vi "Fetch Measurement (Adjacent Channel Power Ratio).vi"(0 "VISA resource name":refnum<visa-resource-name>, 11 "error in (no error)":errorcluster) -> (3 "Main Channel Power(dBm)":dbl, 4 "VISA resource name out":refnum<visa-resource-name>, 6 "Low Adjacent Channel Power(dBm)":dbl[](array[numeric]), 8 "Upper Adjacent Channel Power Ratio(dB)":dbl[](array[numeric]), 10 "Low Adjacent Channel Power Ratio(dB)":dbl[](array[numeric]), 14 "Upper Adjacent Channel Power(dBm)":dbl[](array[numeric]), 15 "error out":errorcluster)   [LabVIEW 2022 SP3, in "Agilent N934X Series.lvlib"]
doc: "Returns the results of last measurement (Adjacent Channel Power Ratio) and does not initiate data acquisition.\n\nNote:\n\nThis VI does not check the instrument status. Typically, you call this VI only in a sequence of calls to other low-level instrument driver VIs. The sequence performs one operation. You use the low-level VIs to optimize one or more aspects of interaction with the instrument. If you want to check the instrument status, call the <B>Error Query VI</B> at the conclusion of the sequence."
uses:
  <instrlib>/Agilent N934X Series/Agilent N934X Series.lvlib
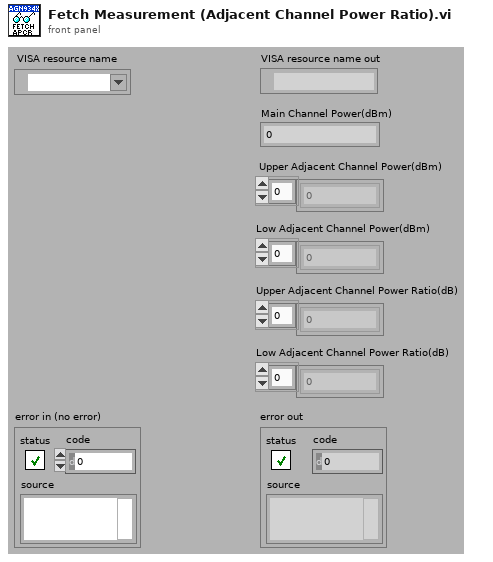
[diagram p1: front panel]
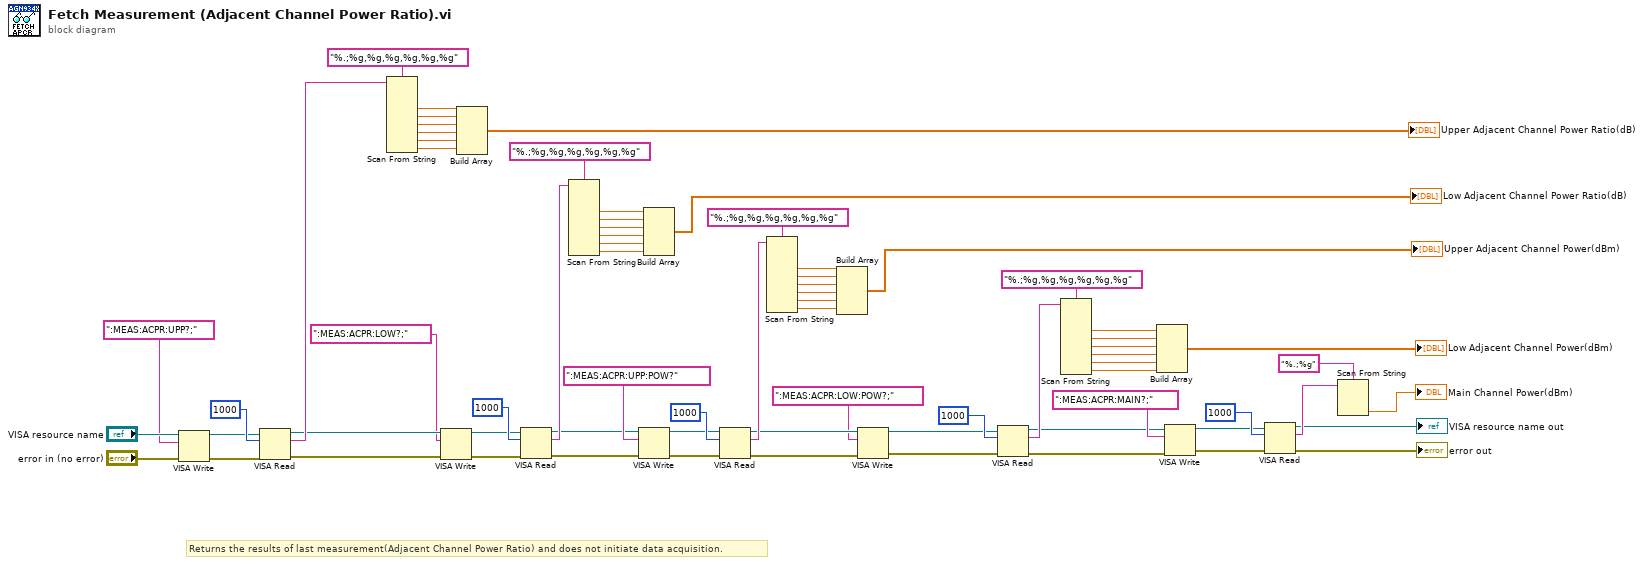
[diagram p0: block diagram]
diagram:
  # "Returns the results of last measurement(Adjacent Channel Power Ratio) and does not initiate data acquisition."
  n1 = VISA Write(VISA resource name="VISA resource name", write buffer=":MEAS:ACPR:UPP?;", error in (no error)="error in (no error)") -> (VISA resource name out=w66:refnum<visa-resource-name>, error out=w65:errorcluster)  [unwired: 1 out]
  n2 = VISA Read(VISA resource name=w66, byte count=u32 1000, error in (no error)=w65) -> (VISA resource name out=w52:refnum<visa-resource-name>, read buffer=w67:string, error out=w51:errorcluster)  [unwired: 1 out]
  n3 = Scan From String(format string="%.;%g,%g,%g,%g,%g,%g", input string=w67) -> (output 1=w64:dbl, output 2=w63:dbl, output 3=w62:dbl, output 4=w61:dbl, output 5=w59:dbl, output 6=w60:dbl)  [unwired: 8 in, 3 out]
  n4 = VISA Write(VISA resource name=w52, write buffer=":MEAS:ACPR:LOW?;", error in (no error)=w51) -> (VISA resource name out=w54:refnum<visa-resource-name>, error out=w53:errorcluster)  [unwired: 1 out]
  n5 = Build Array(w64, w63, w62, w61, w59, w60) -> (→"Upper Adjacent Channel Power Ratio(dB)":dbl[])
  n6 = VISA Read(VISA resource name=w54, byte count=u32 1000, error in (no error)=w53) -> (VISA resource name out=w34:refnum<visa-resource-name>, read buffer=w55:string, error out=w33:errorcluster)  [unwired: 1 out]
  n7 = Scan From String(format string="%.;%g,%g,%g,%g,%g,%g", input string=w55) -> (output 1=w49:dbl, output 2=w50:dbl, output 3=w48:dbl, output 4=w47:dbl, output 5=w46:dbl, output 6=w45:dbl)  [unwired: 8 in, 3 out]
  n8 = VISA Write(VISA resource name=w34, write buffer=":MEAS:ACPR:UPP:POW?", error in (no error)=w33) -> (VISA resource name out=w15:refnum<visa-resource-name>, error out=w16:errorcluster)  [unwired: 1 out]
  n9 = Build Array(w49, w50, w48, w47, w46, w45) -> (→"Low Adjacent Channel Power Ratio(dB)":dbl[])
  n10 = VISA Read(VISA resource name=w15, byte count=u32 1000, error in (no error)=w16) -> (VISA resource name out=w23:refnum<visa-resource-name>, read buffer=w42:string, error out=w22:errorcluster)  [unwired: 1 out]
  n11 = Scan From String(format string="%.;%g,%g,%g,%g,%g,%g", input string=w42) -> (output 1=w41:dbl, output 2=w40:dbl, output 3=w39:dbl, output 4=w38:dbl, output 5=w36:dbl, output 6=w37:dbl)  [unwired: 8 in, 3 out]
  n12 = Build Array(w41, w40, w39, w38, w36, w37) -> (→"Upper Adjacent Channel Power(dBm)":dbl[])
  n13 = VISA Write(VISA resource name=w23, write buffer=":MEAS:ACPR:LOW:POW?;", error in (no error)=w22) -> (VISA resource name out=w14:refnum<visa-resource-name>, error out=w13:errorcluster)  [unwired: 1 out]
  n14 = VISA Read(VISA resource name=w14, byte count=u32 1000, error in (no error)=w13) -> (VISA resource name out=w8:refnum<visa-resource-name>, read buffer=w30:string, error out=w7:errorcluster)  [unwired: 1 out]
  n15 = Scan From String(format string="%.;%g,%g,%g,%g,%g,%g", input string=w30) -> (output 1=w29:dbl, output 2=w28:dbl, output 3=w27:dbl, output 4=w26:dbl, output 5=w24:dbl, output 6=w25:dbl)  [unwired: 8 in, 3 out]
  n16 = Build Array(w29, w28, w27, w26, w24, w25) -> (→"Low Adjacent Channel Power(dBm)":dbl[])
  n17 = VISA Write(VISA resource name=w8, write buffer=":MEAS:ACPR:MAIN?;", error in (no error)=w7) -> (VISA resource name out=w10:refnum<visa-resource-name>, error out=w9:errorcluster)  [unwired: 1 out]
  n18 = VISA Read(VISA resource name=w10, byte count=u32 1000, error in (no error)=w9) -> (VISA resource name out=→"VISA resource name out":refnum<visa-resource-name>, read buffer=w5:string, error out=→"error out":errorcluster)  [unwired: 1 out]
  n19 = Scan From String(format string="%.;%g", input string=w5) -> (output 1=→"Main Channel Power(dBm)":dbl)  [unwired: 3 in, 3 out]
